vi "5.vi"(8 "error constant":errorcluster, 11 "Hexahedron":T1={"First base's length of trapezoid"=1.0, "Second base's length of trapezoid"=1.0, " Height of trapezoid"=1.0, "Leg's length of trapezoid"=1.0, "Hexahedron's height"=1.0} {"Hexahedron's height" min=1e-10; "Leg's length of trapezoid" min=1e-10; "Height of trapezoid" min=1e-10; "Second base's length of trapezoid" min=1e-10; "First base's length of trapezoid" min=1e-10}) -> (0 "error constant 2":errorcluster, 3 "Area":dbl)   [LabVIEW 2020]
doc: "Return area of hexahedron (inputs, correct order --> length of: two bases of trapezoid; height of trapezoid, length of leg of trapezoid, height of hexahedron)"
uses:
  AreaOfHexahedron.ctl
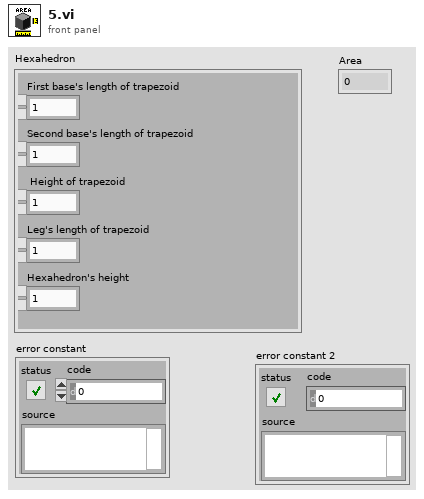
[diagram p1: front panel]
types:
  T1 = typedef "AreaOfHexahedron.ctl" = cluster{"First base's length of trapezoid":dbl, "Second base's length of trapezoid":dbl, " Height of trapezoid":dbl, "Leg's length of trapezoid":dbl, "Hexahedron's height":dbl}
  T2 = cluster{"First base's length of trapezoid":bool, "Second base's length of trapezoid":bool, " Height of trapezoid":bool, "Leg's length of trapezoid":bool, "Hexahedron's height":bool}
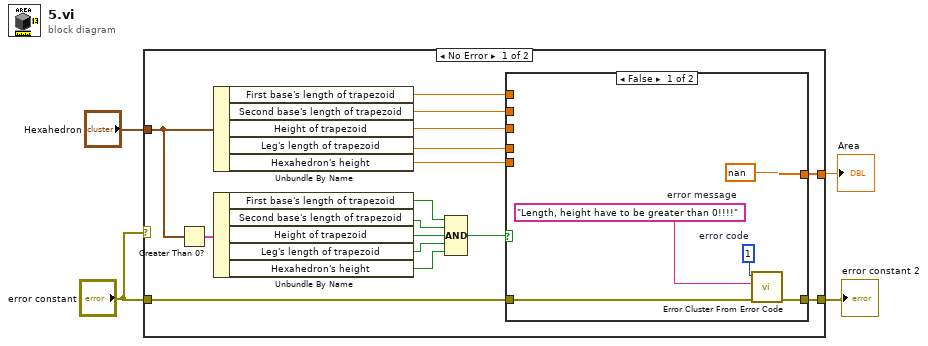
[diagram p0: block diagram]
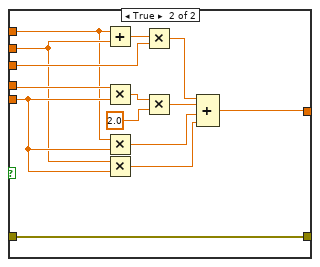
[diagram p2: hidden frame]
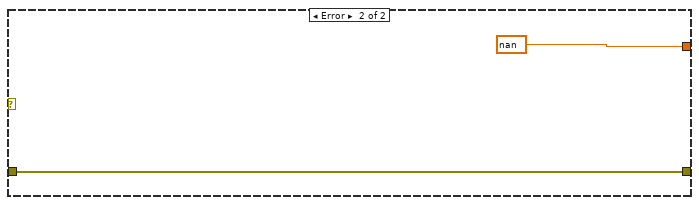
[diagram p3: hidden frame]
diagram:
  n1 = case shown="No Error" "error constant" {
    tunnel: [w20 nan] -> w4
    tunnel: "Hexahedron" -> [w14 _]
    tunnel: "error constant" -> [w6 w41]
    tunnel: [w5 w41] -> w1
    frame No Error {
      n2 = Greater Than 0?(x=w14) -> (x > 0?=w13:T2)
      n3 = Unbundle By Name(w14) -> ("First base's length of trapezoid"=w15:dbl, "Second base's length of trapezoid"=w16:dbl, "Height of trapezoid"=w17:dbl, "Leg's length of trapezoid"=w18:dbl, "Hexahedron's height"=w19:dbl)
      n4 = Unbundle By Name(w13) -> ("First base's length of trapezoid"=w12:bool, "Second base's length of trapezoid"=w11:bool, "Height of trapezoid"=w10:bool, "Leg's length of trapezoid"=w9:bool, "Hexahedron's height"=w8:bool)
      n5 = Compound Arithmetic op=AND(w12, w11, w10, w9, w8) -> (w7:bool)
      n6 = case shown="False" w7 {
        tunnel: [nan w39] -> w20
        tunnel: w19 -> [_ w38]
        tunnel: w18 -> [_ w37]
        tunnel: w17 -> [_ w36]
        tunnel: w16 -> [_ w35]
        tunnel: w15 -> [_ w34]
        tunnel: w6 -> [w23 w26]
        tunnel: [w22 w26] -> w5
        frame False {
          w21 = "Length, height have to be greater than 0!!!!"  # error message
          w24 = 1  # error code
          n7 = call <vilib>:"Error Cluster From Error Code.vi"("error in (no error)"=w23, "error message (\"\")"=w21, "error code (0)"=w24) -> ("error out"=w22:errorcluster)  [unwired: 6 in]
        }
        frame True {
          n8 = Add(x=w34, y=w35) -> (x+y=w33:dbl)
          n9 = Multiply(x=w37, y=w38) -> (x*y=w32:dbl)
          n10 = Multiply(x=w34, y=w38) -> (x*y=w28:dbl)
          n11 = Multiply(x=w35, y=w38) -> (x*y=w27:dbl)
          n12 = Multiply(x=w33, y=w36) -> (x*y=w30:dbl)
          n13 = Multiply(x=w32, y=2.0) -> (x*y=w29:dbl)
          n14 = Compound Arithmetic op=ADD(w30, w29, w28, w27) -> (w39:dbl)
        }
      }
    }
    frame Error {
    }
  }
  "Area" <- w4
  "error constant 2" <- w1
